vi "加标回收启动 (子VI).vi"(11 "启动参数":T1(ring)=enum."CODCr") -> (0 "error out":T2={"status"=FALSE, "代码"=4, "source"=""} caption="错误输出" {"代码" items=["执行成功"=1, "执行失败，但不知道原因"=2, "命令请求条件错误"=3, "通讯超时"=4, "系统繁忙不能执行"=5, "系统故障"=6, "没有数据"=100]})   [LabVIEW 2016]
uses:
  PLC/PLC.lvlib
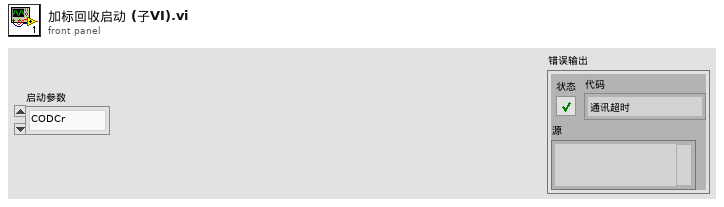
[diagram p1: front panel]
types:
  T1 = enum16{"未选择", "CODMn", "氨氮", "总磷", "总氮", "CODCr"}
  T2 = cluster{"status":bool, "代码":u16, "source":string}
  T3 = enum16{"空闲", "水样测试", "标样核查", "零点核查", "跨度核查", "空白测试", "平行样测试", "质控样", "空白校准", "标样校准", "加标回收"}
  T4 = enum16{"空闲", "水样测试", "标样核查", "零点核查", "跨度核查", "空白测试", "平行样测试", "加标回收", "空白校准", "标样校准", "初始化（清洗）"}
  T5 = cluster{"R0":i16, "R1":i16, "R2":i16, "R3":i16, "R4":i16, "R5":i16, "R6":i16, "R7":i16, "R8":i16, "R9":i16, "R10":i16, "R11":i16, "R12":i16, "R13":i16, "R14":i16, "R15":i16, "R16":i16, "R17":i16, "R18":i16, "R19":i16, "R20":i16, "R21":i16, "R22":i16, "R23":i16, "R24":i16, "R25":i16, "R26":i16, "R27":i16, "R28":i16, "R29":i16, "R30":i16, "R31":i16, "R32":i16, "R33":i16, "R34":i16, "R35":i16, "R36":i16, "R37":i16, "R38":i16, "R39":i16}
  T6 = enum32{"Bad", "Idle", "Run top level", "Running"}
  T7 = cluster{"系统时间":timestamp, "工作状态":enum16{"空闲", "水样测试", "标样核查", "零点核查", "跨度核查", "空白测试", "平行样测试", "加标回收", "空白校准", "标样校准", "初始化（清洗）"}, "测量模式":enum16{"待机", "连续模式", "周期模式", "定点模式", "受控模式", "手动模式"}, "告警代码":u16, "故障代码":u16, "日志代码":u16, "软件版本":u16, "F0":sgl, "F1":sgl, "F2":sgl, "F3":sgl, "T":sgl, "H":sgl, "id":u16, "flowid":u16, "量程":u16, "总磷控温温度1":sgl, "营养盐控温温度2":sgl, "ADC":sgl}
  T8 = cluster{"系统时间":timestamp, "工作状态":u16, "测量模式":u16, "告警代码":u16, "故障代码":u16, "日志代码":u16, "软件版本":u16, "F0":sgl, "F1":sgl, "F2":sgl, "F3":sgl, "T":sgl, "H":sgl, "id":u16, "flowid":u16, "量程":u16}
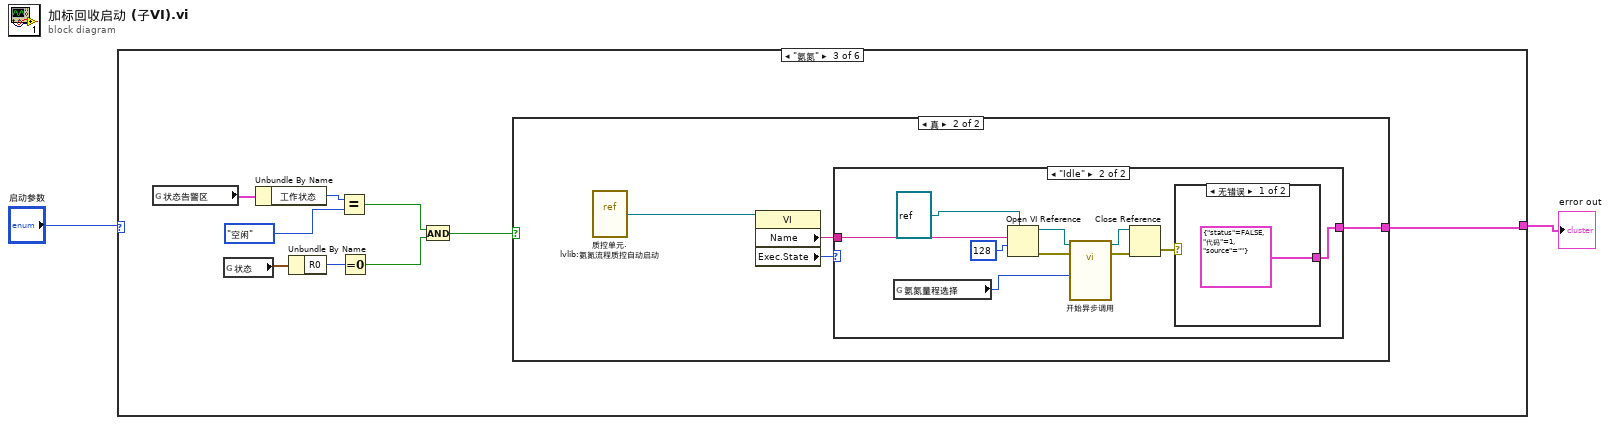
[diagram p0: block diagram]
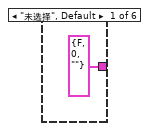
[diagram p2: hidden frame]
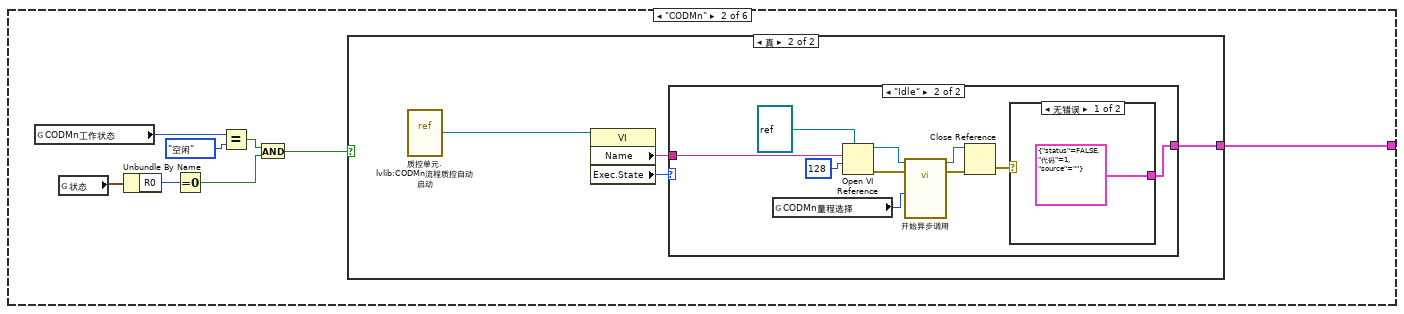
[diagram p3: hidden frame]
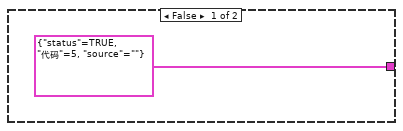
[diagram p4: hidden frame]
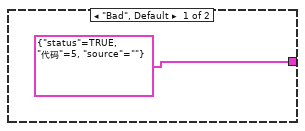
[diagram p5: hidden frame]
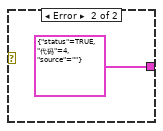
[diagram p6: hidden frame]
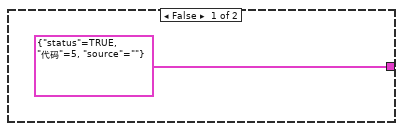
[diagram p7: hidden frame]
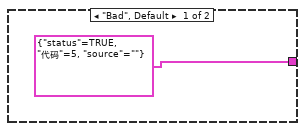
[diagram p8: hidden frame]
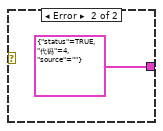
[diagram p9: hidden frame]
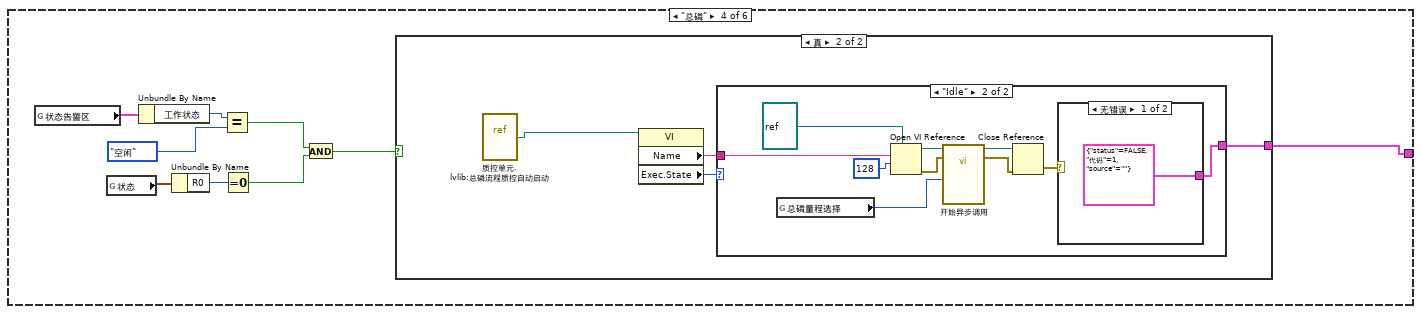
[diagram p10: hidden frame]
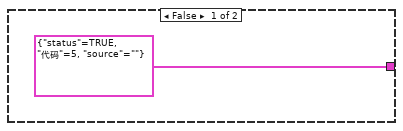
[diagram p11: hidden frame]
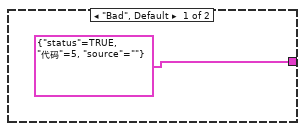
[diagram p12: hidden frame]
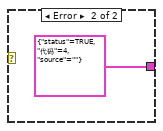
[diagram p13: hidden frame]
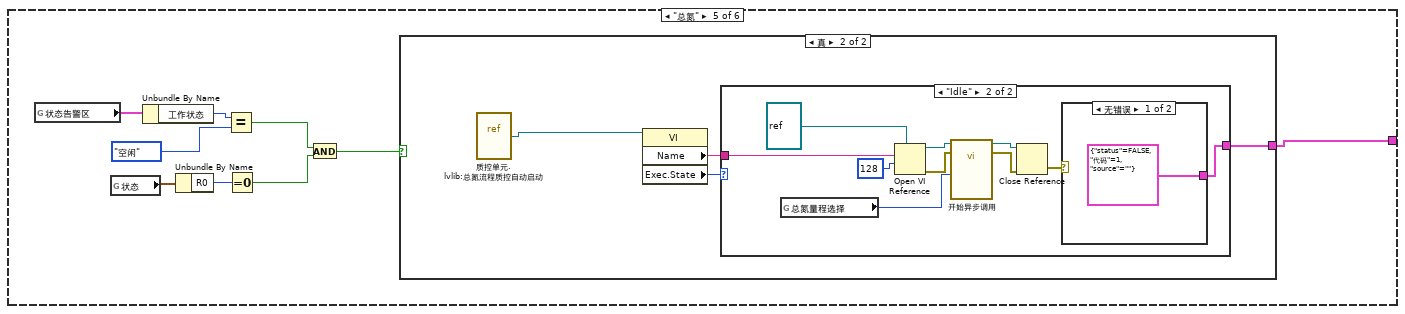
[diagram p14: hidden frame]
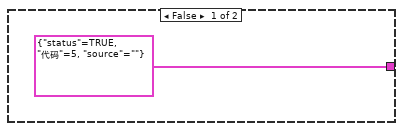
[diagram p15: hidden frame]
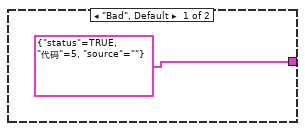
[diagram p16: hidden frame]
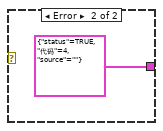
[diagram p17: hidden frame]
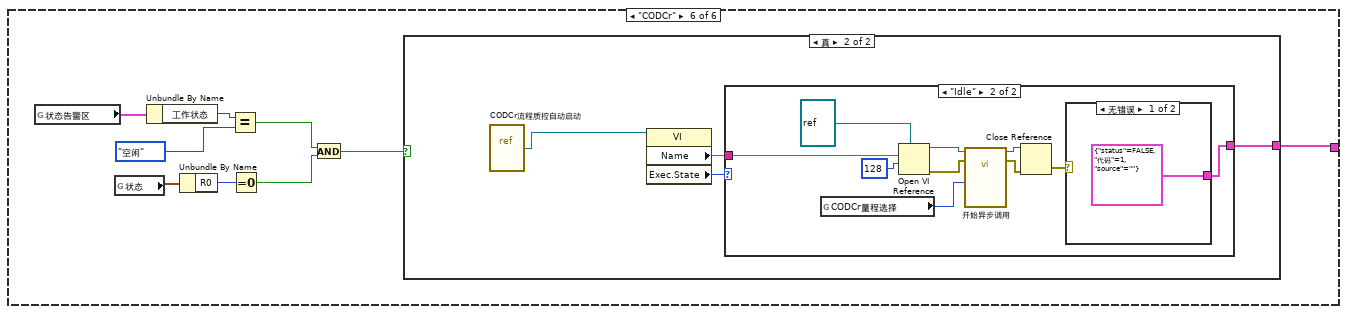
[diagram p18: hidden frame]
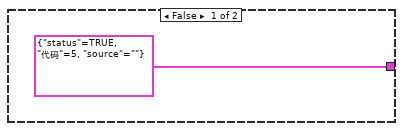
[diagram p19: hidden frame]
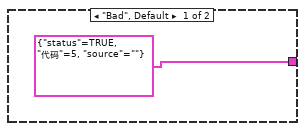
[diagram p20: hidden frame]
diagram:
  n1 = case shown="\"氨氮\"" "启动参数" {
    tunnel: [T2 {"status"=FALSE, "代码"=0, "source"=""} ("error out") w4 w34 w58 w84 w112] -> w1
    frame "未选择", Default {
    }
    frame "CODMn" {
      n2 = global read "COD测量模式全局.vi" "CODMn工作状态"() -> (w11:T3)
      n3 = global read "采配水全局变量.vi" "状态"() -> (w8:T5)
      n4 = Unbundle By Name(w8) -> ("R0"=w7:i16)
      n5 = Equal To 0?(x=w7) -> (x = 0?=w6:bool)
      n6 = Equal?(x=w11, y=T3."空闲") -> (x = y?=w9:bool)
      n7 = And(x=w9, y=w6) -> (x .and. y?=w5:bool)
      n8 = case shown="真" w5 {
        tunnel: [T2 {"status"=TRUE, "代码"=5, "source"=""} ("error out") w13] -> w4
        frame False {
        }
        frame True {
          n9 = vi-ref "质控单元.lvlib:CODMn流程质控自动启动.vi"() -> (w14:refnum<vi>)
          n10 = property class="VI"(reference=w14) -> ("Name"=w16:string, "Exec.State"=w15:T6)  [unwired: 1 in, 2 out]
          n11 = case shown="\"Idle\"" w15 {
            tunnel: w16 -> [_ w24]
            tunnel: [T2 {"status"=TRUE, "代码"=5, "source"=""} ("error out") w20] -> w13
            frame "Bad", Default {
            }
            frame "Idle" {
              n12 = global read "断电保存全局.vi" "CODMn量程选择"() -> (w18:enum32{"H", "L", "AUTO"})
              n13 = Open VI Reference(type specifier VI Refnum (for type only)=refnum<vi> refnum ("类型说明符VI引用句柄（仅用于类型）"), vi path=w24, options=128 ("选项")) -> (vi reference=w19:refnum<vi>, error out=w23:errorcluster)  [unwired: 3 in]
              n14 = call-by-ref "开始异步调用"(reference=w19, error in=w23, "CODMn量程切换"=w18) -> (reference out=w27:refnum<vi>, error out=w22:errorcluster)  [unwired: 10 in]
              n15 = Close Reference(reference=w27, error in (no error)=w22) -> (error out=w21:errorcluster)
              n16 = case shown="无错误" w21 {
                tunnel: [T2 {"status"=FALSE, "代码"=1, "source"=""} ("error out") T2 {"status"=TRUE, "代码"=4, "source"=""} ("error out")] -> w20
                frame No Error {
                }
                frame Error {
                }
              }
            }
          }
        }
      }
    }
    frame "氨氮" {
      n17 = global read "VAR总磷总氮全局变量.vi" "状态告警区"() -> (w33:T7)
      n18 = global read "采配水全局变量.vi" "状态"() -> (w38:T5)
      n19 = Unbundle By Name(w33) -> ("工作状态"=w32:T4)
      n20 = Unbundle By Name(w38) -> ("R0"=w37:i16)
      n21 = Equal?(x=w32, y=T4."空闲") -> (x = y?=w30:bool)
      n22 = Equal To 0?(x=w37) -> (x = 0?=w36:bool)
      n23 = And(x=w30, y=w36) -> (x .and. y?=w35:bool)
      n24 = case shown="真" w35 {
        tunnel: [T2 {"status"=TRUE, "代码"=5, "source"=""} ("error out") w41] -> w34
        frame False {
        }
        frame True {
          n25 = vi-ref "质控单元.lvlib:氨氮流程质控自动启动.vi"() -> (w40:refnum<vi>)
          n26 = property class="VI"(reference=w40) -> ("Name"=w43:string, "Exec.State"=w42:T6)  [unwired: 1 in, 2 out]
          n27 = case shown="\"Idle\"" w42 {
            tunnel: w43 -> [_ w51]
            tunnel: [T2 {"status"=TRUE, "代码"=5, "source"=""} ("error out") w47] -> w41
            frame "Bad", Default {
            }
            frame "Idle" {
              n28 = global read "断电保存全局.vi" "氨氮量程选择"() -> (w45:enum32{"H", "L", "AUTO"})
              n29 = Open VI Reference(type specifier VI Refnum (for type only)=refnum<vi> refnum ("类型说明符VI引用句柄（仅用于类型）"), vi path=w51, options=128 ("选项")) -> (vi reference=w54:refnum<vi>, error out=w50:errorcluster)  [unwired: 3 in]
              n30 = call-by-ref "开始异步调用"(reference=w54, error in=w50, "氨氮量程切换"=w45) -> (reference out=w53:refnum<vi>, error out=w49:errorcluster)  [unwired: 11 in]
              n31 = Close Reference(reference=w53, error in (no error)=w49) -> (error out=w48:errorcluster)
              n32 = case shown="无错误" w48 {
                tunnel: [T2 {"status"=FALSE, "代码"=1, "source"=""} ("error out") T2 {"status"=TRUE, "代码"=4, "source"=""} ("error out")] -> w47
                frame No Error {
                }
                frame Error {
                }
              }
            }
          }
        }
      }
    }
    frame "总磷" {
      n33 = global read "VAR总磷总氮全局变量.vi" "状态告警区"() -> (w57:T7)
      n34 = global read "采配水全局变量.vi" "状态"() -> (w65:T5)
      n35 = Unbundle By Name(w57) -> ("工作状态"=w61:T4)
      n36 = Unbundle By Name(w65) -> ("R0"=w64:i16)
      n37 = Equal?(x=w61, y=T4."空闲") -> (x = y?=w59:bool)
      n38 = Equal To 0?(x=w64) -> (x = 0?=w63:bool)
      n39 = And(x=w59, y=w63) -> (x .and. y?=w62:bool)
      n40 = case shown="真" w62 {
        tunnel: [T2 {"status"=TRUE, "代码"=5, "source"=""} ("error out") w68] -> w58
        frame False {
        }
        frame True {
          n41 = vi-ref "质控单元.lvlib:总磷流程质控自动启动.vi"() -> (w67:refnum<vi>)
          n42 = property class="VI"(reference=w67) -> ("Name"=w70:string, "Exec.State"=w69:T6)  [unwired: 1 in, 2 out]
          n43 = case shown="\"Idle\"" w69 {
            tunnel: w70 -> [_ w80]
            tunnel: [T2 {"status"=TRUE, "代码"=5, "source"=""} ("error out") w77] -> w68
            frame "Bad", Default {
            }
            frame "Idle" {
              n44 = global read "断电保存全局.vi" "总磷量程选择"() -> (w72:enum32{"H", "L", "AUTO"})
              n45 = Open VI Reference(type specifier VI Refnum (for type only)=refnum<vi> refnum ("类型说明符VI引用句柄（仅用于类型）"), vi path=w80, options=128 ("选项")) -> (vi reference=w75:refnum<vi>, error out=w74:errorcluster)  [unwired: 3 in]
              n46 = call-by-ref "开始异步调用"(reference=w75, error in=w74, "总磷量程切换"=w72) -> (reference out=w73:refnum<vi>, error out=w79:errorcluster)  [unwired: 11 in]
              n47 = Close Reference(reference=w73, error in (no error)=w79) -> (error out=w78:errorcluster)
              n48 = case shown="无错误" w78 {
                tunnel: [T2 {"status"=FALSE, "代码"=1, "source"=""} ("error out") T2 {"status"=TRUE, "代码"=4, "source"=""} ("error out")] -> w77
                frame No Error {
                }
                frame Error {
                }
              }
            }
          }
        }
      }
    }
    frame "总氮" {
      n49 = global read "VAR总磷总氮全局变量.vi" "状态告警区"() -> (w85:T7)
      n50 = global read "采配水全局变量.vi" "状态"() -> (w92:T5)
      n51 = Unbundle By Name(w85) -> ("工作状态"=w88:T4)
      n52 = Unbundle By Name(w92) -> ("R0"=w91:i16)
      n53 = Equal?(x=w88, y=T4."空闲") -> (x = y?=w86:bool)
      n54 = Equal To 0?(x=w91) -> (x = 0?=w90:bool)
      n55 = And(x=w86, y=w90) -> (x .and. y?=w89:bool)
      n56 = case shown="真" w89 {
        tunnel: [T2 {"status"=TRUE, "代码"=5, "source"=""} ("error out") w95] -> w84
        frame False {
        }
        frame True {
          n57 = vi-ref "质控单元.lvlib:总氮流程质控自动启动.vi"() -> (w94:refnum<vi>)
          n58 = property class="VI"(reference=w94) -> ("Name"=w97:string, "Exec.State"=w96:T6)  [unwired: 1 in, 2 out]
          n59 = case shown="\"Idle\"" w96 {
            tunnel: w97 -> [_ w107]
            tunnel: [T2 {"status"=TRUE, "代码"=5, "source"=""} ("error out") w105] -> w95
            frame "Bad", Default {
            }
            frame "Idle" {
              n60 = global read "断电保存全局.vi" "总氮量程选择"() -> (w101:enum32{"H", "L", "AUTO"})
              n61 = Open VI Reference(type specifier VI Refnum (for type only)=refnum<vi> refnum ("类型说明符VI引用句柄（仅用于类型）"), vi path=w107, options=128 ("选项")) -> (vi reference=w103:refnum<vi>, error out=w102:errorcluster)  [unwired: 3 in]
              n62 = call-by-ref "开始异步调用"(reference=w103, error in=w102, "总氮量程切换"=w101) -> (reference out=w100:refnum<vi>, error out=w99:errorcluster)  [unwired: 11 in]
              n63 = Close Reference(reference=w100, error in (no error)=w99) -> (error out=w106:errorcluster)
              n64 = case shown="无错误" w106 {
                tunnel: [T2 {"status"=FALSE, "代码"=1, "source"=""} ("error out") T2 {"status"=TRUE, "代码"=4, "source"=""} ("error out")] -> w105
                frame No Error {
                }
                frame Error {
                }
              }
            }
          }
        }
      }
    }
    frame "CODCr" {
      n65 = global read "CODcr全局变量.vi" "状态告警区"() -> (w111:T8)
      n66 = global read "采配水全局变量.vi" "状态"() -> (w119:T5)
      n67 = Unbundle By Name(w111) -> ("工作状态"=w115:u16)
      n68 = Unbundle By Name(w119) -> ("R0"=w118:i16)
      n69 = Equal?(x=w115, y=T4."空闲") -> (x = y?=w113:bool)
      n70 = Equal To 0?(x=w118) -> (x = 0?=w117:bool)
      n71 = And(x=w113, y=w117) -> (x .and. y?=w116:bool)
      n72 = case shown="真" w116 {
        tunnel: [T2 {"status"=TRUE, "代码"=5, "source"=""} ("error out") w122] -> w112
        frame False {
        }
        frame True {
          n73 = vi-ref "CODCr流程质控自动启动.vi"() -> (w121:refnum<vi>)
          n74 = property class="VI"(reference=w121) -> ("Name"=w124:string, "Exec.State"=w123:T6)  [unwired: 1 in, 2 out]
          n75 = case shown="\"Idle\"" w123 {
            tunnel: w124 -> [_ w134]
            tunnel: [T2 {"status"=TRUE, "代码"=5, "source"=""} ("error out") w132] -> w122
            frame "Bad", Default {
            }
            frame "Idle" {
              n76 = global read "断电保存全局.vi" "CODCr量程选择"() -> (w129:enum32{"H", "L", "AUTO"})
              n77 = Open VI Reference(type specifier VI Refnum (for type only)=refnum<vi> refnum ("类型说明符VI引用句柄（仅用于类型）"), vi path=w134, options=128 ("选项")) -> (vi reference=w130:refnum<vi>, error out=w128:errorcluster)  [unwired: 3 in]
              n78 = call-by-ref "开始异步调用"(reference=w130, error in=w128, "CODCr量程切换"=w129) -> (reference out=w127:refnum<vi>, error out=w126:errorcluster)  [unwired: 10 in]
              n79 = Close Reference(reference=w127, error in (no error)=w126) -> (error out=w133:errorcluster)
              n80 = case shown="无错误" w133 {
                tunnel: [T2 {"status"=FALSE, "代码"=1, "source"=""} ("error out") T2 {"status"=TRUE, "代码"=4, "source"=""} ("error out")] -> w132
                frame No Error {
                }
                frame Error {
                }
              }
            }
          }
        }
      }
    }
  }
  "error out" <- w1
